vi "Normalize.vi"(1 "limite basse":dbl, 2 "limite haute":dbl, 3 "Input Array":dbl[](array[numeric])) -> (0 "normailzed array 2":dbl[](array[numeric]))   [LabVIEW 2011]
panel:
  out "normailzed array 1":dbl[](array[numeric])
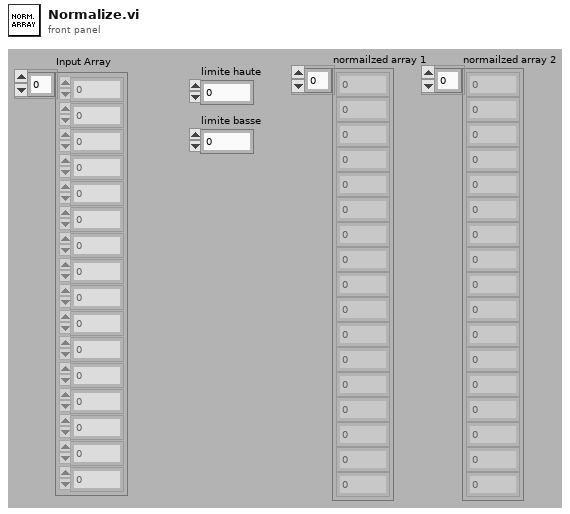
[diagram p1: front panel]
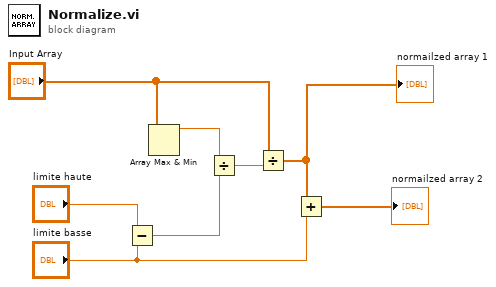
[diagram p0: block diagram]
diagram:
  n1 = Subtract(x="limite haute", y="limite basse") -> (x-y=w6:dbl)
  n2 = Array Max & Min(array="Input Array") -> (max value=w7:dbl)  [unwired: 3 out]
  n3 = Divide(x=w7, y=w6) -> (x/y=w4:dbl)
  n4 = Divide(x="Input Array", y=w4) -> (x/y=w3:dbl[])
  "normailzed array 1" <- w3
  n5 = Add(x=w3, y="limite basse") -> (x+y=→"normailzed array 2":dbl[])
